vi "Delete Element at End.vi"(8 "error in (no error)":errorcluster, 11 "Variant in":variant) -> (0 "error out":errorcluster, 3 "Variant out":variant, 9 "element":variant, 10 "Name":string)   [LabVIEW 2017, in "Advanced Variant Tools.lvlib" / "Cluster Manipulation.lvlib"]
uses:
  Cluster Manipulation.lvlib
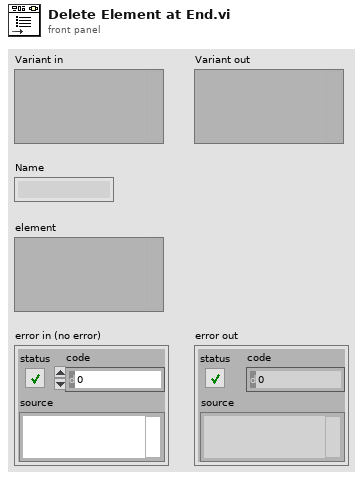
[diagram p1: front panel]
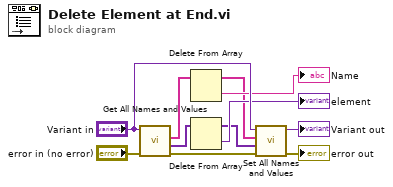
[diagram p0: block diagram]
diagram:
  n1 = call "Get All Names and Values.vi"("error in"="error in (no error)", "Cluster In"="Variant in") -> ("error out"=w9:errorcluster, "Values"=w10:variant[], "Names"=w5:string[])  [unwired: 6 in, 1 out]
  n2 = Delete From Array(array=w5) -> (deleted portion=→"Name":string, array with subset deleted=w2:string[])  [unwired: 2 in]
  n3 = Delete From Array(array=w10) -> (deleted portion=→"element":variant, array with subset deleted=w1:variant[])  [unwired: 2 in]
  n4 = call "Set All Names and Values.vi"("error in"=w9, "values"=w1, "Names"=w2, "Cluster In"="Variant in") -> ("error out"=→"error out":errorcluster, "Cluster Out"=→"Variant out":variant)  [unwired: 6 in]
